vi "Find By GUID.vi"(10 "GUID":u16) -> (2 "Found?":bool, 3 "Team":T1)   [LabVIEW 2013]
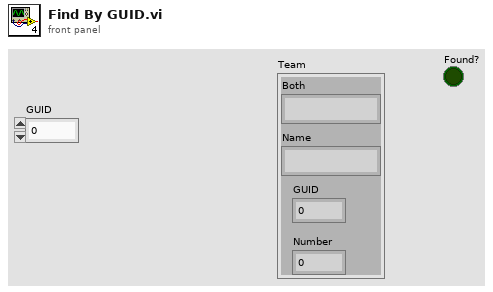
[diagram p1: front panel]
types:
  T1 = cluster{"Both":string, "Name":string, "GUID":u16, "Number":u16}
  T2 = enum16{"Get Teams", "Add Team", "Modify Team", "Clear All Teams", "Force Add Team", "Delete Team"}
  T3 = typedef "Team Data.ctl" = cluster{"Both":string, "Name":string, "GUID":u16, "Number":u16}
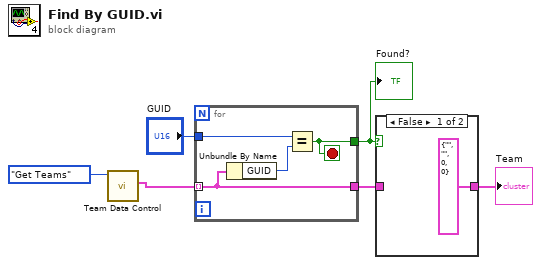
[diagram p0: block diagram]
diagram:
  n1 = call "Team Data Control.vi"("Mode"=T2."Get Teams") -> ("Team Array Out"=w1:T3[])  [unwired: 10 in]
  n2 = for {
    tunnel: w1 -> [w8] mode=indexing
    tunnel: "GUID" -> [w9]
    tunnel: [w8] -> w4
    tunnel: [w7] -> w5
    stop <- w7 stop-if-true
    n3 = Unbundle By Name(w8) -> ("GUID"=w10:u16)
    n4 = Equal?(x=w9, y=w10) -> (x = y?=w7:bool)
  }
  "Found?" <- w5
  n5 = case shown="False" w5 {
    tunnel: [T1 {"Both"="", "Name"="", "GUID"=0, "Number"=0} w12] -> w3
    tunnel: w4 -> [_ w12]
    frame False {
    }
    frame True {
    }
  }
  "Team" <- w3
